vi "Get Node (Extended).vi"(8 "error in (no error)":errorcluster, 10 "Node":string, 11 "Test Result in":refnum<class "Test Result.lvclass">) -> (0 "error out":errorcluster, 1 "Assertions":T3[](array[typedef]), 2 "Test Node":T1, 3 "Test Result out":refnum<class "Test Result.lvclass">, 4 "found":bool, 5 "indent level":i32)   [LabVIEW 2020, in "Caraya.lvlib" / "Test Result.lvclass"]
uses:
  Test Result.lvclass
  Assert Event Data (Extended).ctl
  Test Node (Extended).ctl
  Test Registration Data.ctl
  Test Result.lvclass/Test Result.ctl
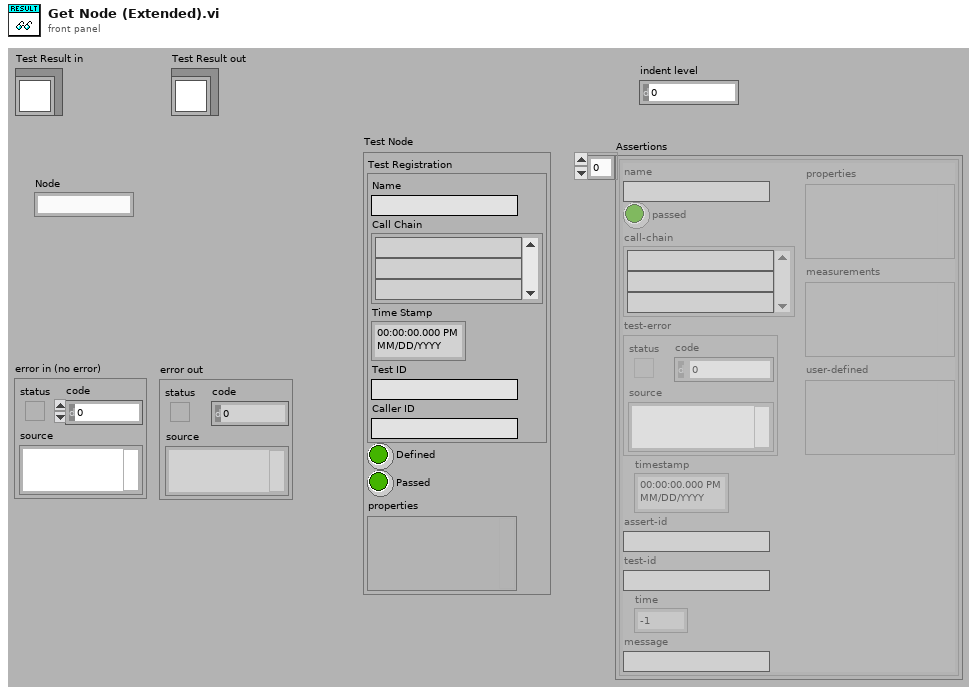
[diagram p1: front panel]
types:
  T1 = typedef "Caraya.lvlib/Test Result.lvclass/Test Node (Extended).ctl" = cluster{"Test Registration":T2, "Defined":bool, "Passed":bool, "properties":variant}
  T2 = typedef "Caraya.lvlib/Test Result.lvclass/Test Registration Data.ctl" = cluster{"Name":string, "Call Chain":string[], "Time Stamp":timestamp, "Test ID":string, "Caller ID":string}
  T3 = typedef "Caraya.lvlib/Test Result.lvclass/Assert Event Data (Extended).ctl" = cluster{"name":string, "passed":bool, "call-chain":string[], "test-error":errorcluster, "timestamp":timestamp, "assert-id":string, "test-id":string, "time":dbl, "message":string, "properties":variant, "measurements":variant, "user-defined":variant}
  T4 = typedef "Caraya.lvlib/Test Result.lvclass/Node Results (Extended).ctl" = cluster{"Test Node":T1, "Assertions":T3[]}
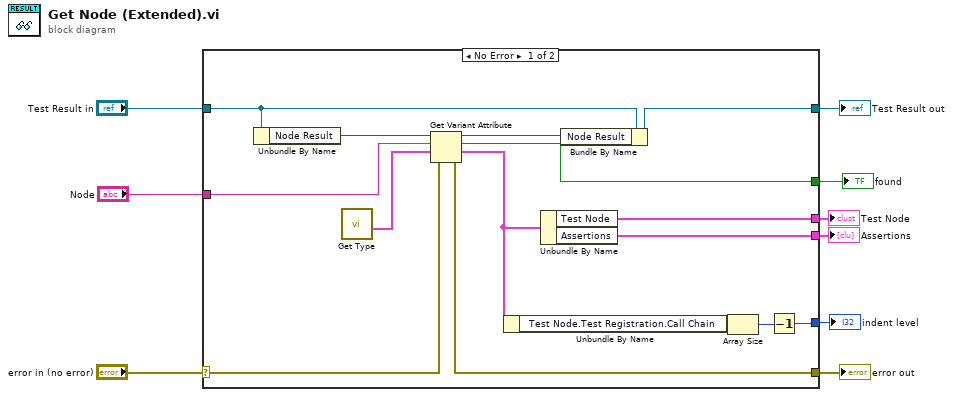
[diagram p0: block diagram]
diagram:
  n1 = case shown="No Error" "error in (no error)" {
    selector: "error in (no error)" -> [w19 w26]
    tunnel: [w20 w26] -> w8
    tunnel: [w23 w25] -> w6
    tunnel: "Test Result in" -> [w24 w25]
    tunnel: "Node" -> [w18 _]
    tunnel: [w17 _] -> w4
    tunnel: [w16 _] -> w2
    tunnel: [w10 _] -> w3
    tunnel: [w12 _] -> w1
    frame No Error {
      n2 = Unbundle By Name(w24) -> ("Node Result"=w22:variant)
      n3 = call "Get Type.vi"() -> ("Extended Node Result"=w11:T4)  [unwired: 10 in, 1 out]
      n4 = Get Variant Attribute(Variant=w22, name=w18, default value (empty Variant)=w11, error in=w19) -> (duplicate Variant=w21:variant, found=w17:bool, value=w15:T4, error out=w20:errorcluster)
      n5 = Unbundle By Name(w15) -> ("Test Node.Test Registration.Call Chain"=w14:string[])
      n6 = Unbundle By Name(w15) -> ("Test Node"=w16:T1, "Assertions"=w10:T3[])
      n7 = Bundle By Name(cluster=w24, "Node Result"=w21) -> (w23:refnum<class "Test Result.lvclass">)
      n8 = Array Size(array=w14) -> (size(s)=w13:i32)
      n9 = Decrement(x=w13) -> (x-1=w12:i32)
    }
    frame Error {
    }
  }
  "error out" <- w8
  "Test Result out" <- w6
  "found" <- w4
  "Assertions" <- w3
  "Test Node" <- w2
  "indent level" <- w1
